vi "ini配置文件读取（I32）.vi"(9 "key":string caption="键", 10 "section":string caption="段", 11 "文件名称":string="配置文件") -> (3 "value":i32 caption="值")   [LabVIEW 2018]
uses:
  <vilib>/Utility/error.llb/DialogType.ctl
  <vilib>/Utility/config.llb/Read Key (I32).vi
  <vilib>/Utility/config.llb/NI_LVConfig.lvlib
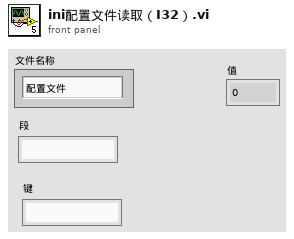
[diagram p1: front panel]
types:
  T1 = typedef "DialogType.ctl" = u16
  T2 = typedef "NI_LVConfig.lvlib/Config Data RefNum.ctl" = refnum<k1>
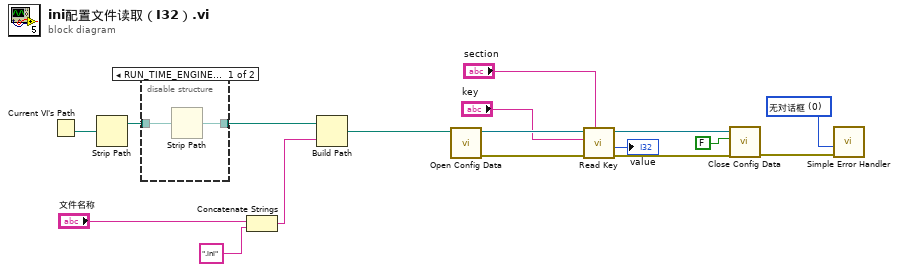
[diagram p0: block diagram]
diagram:
  w8 = T1 0 items=["无对话框", "确定信息", "继续或停止信息", "确定信息＋警告", "继续/停止+警告"] ("type of dialog (OK msg:1)")
  n1 = Current VI's Path() -> (path=w16:path)
  n2 = Strip Path(path=w16) -> (stripped path=w15:path)  [unwired: 1 out]
  n3 = disable-structure shown="RUN_TIME_ENGINE==True" {
    disable-tunnel: w15 -> [w19 w20]
    disable-tunnel: [w18 w20] -> w14
    frame condition #0 {
      n4 = Strip Path(path=w19) -> (stripped path=w18:path)  [unwired: 1 out]
    }
    frame condition #1 (active) {
    }
  }
  n5 = Concatenate Strings("文件名称", ".ini" ("字符串")) -> (w12:string)
  n6 = Build Path(base path=w14, name or relative path=w12) -> (appended path=w17:path)
  n7 = call <vilib>:"Open Config Data.vi"("configuration file path"=w17) -> ("error out"=w3:errorcluster, "refnum"=w6:T2)  [unwired: 2 in, 7 out]
  n8 = call-poly <vilib>:"Read Key.vi"("section"="section", "error in (no error)"=w3, "key"="key", "refnum"=w6) -> ("error out"=w7:errorcluster, "value"=→"value":i32, "refnum out"=w2:T2)  [unwired: 1 in, 4 out]
  n9 = call <vilib>:"Close Config Data.vi"("error in (no error)"=w7, "write file if changed (T)"=FALSE ("write configuration file? (T)"), "refnum"=w2) -> ("error out"=w9:errorcluster)  [unwired: 8 out]
  n10 = call <vilib>:"Simple Error Handler.vi"("type of dialog (OK msg:1)"=w8, "error in (no error)"=w9) -> ()  [unwired: 8 out]
